vi "CollimationLightScan.vi"(6 "Backgrund":T1, 7 "Session In":T2, 10 "扫描范围":dbl) -> (2 "近场准直图像":T1(plugin-control))   [LabVIEW 2018]
uses:
  <vilib>/userdefined/High Color/IMAQdx.ctl
  <vilib>/vision/Image Controls.llb/IMAQ Image.ctl
  <vilib>/vision/NI_Vision_Development_Module.lvlib
  <vilib>/vision/driver/NI_Vision_Acquisition_Software.lvlib
  <resource>/objmgr/IMAQImage.rc
panel:
  out "offset":i32[](array[numeric])
  in  "停止":bool
  out "进度":dbl format="%05.2f%"
  out "YResolution":i32
  out "X Resolution":i32
  out "采集时间":u32
  out "运动时间":u32
  out "总时间":u32
  out "单步时间":u32
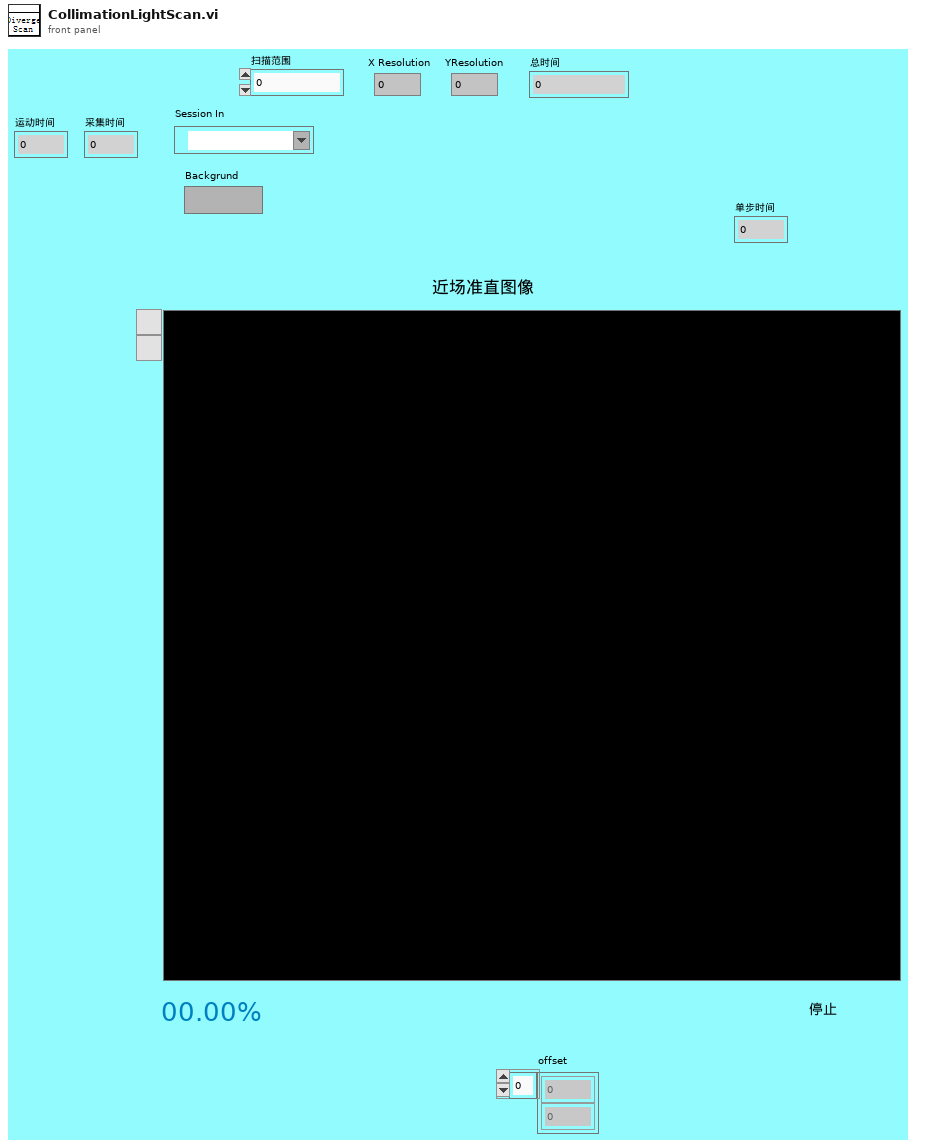
[diagram p1: front panel]
types:
  T1 = typedef "IMAQ Image.ctl" = refnum<image>
  T2 = typedef "IMAQdx.ctl" = refnum<k21>
  T3 = typedef "Image Type" = u32
  T4 = typedef "控制电机位置枚举器.ctl" = enum16{"远场扫描", "发散角扫描", "远场相机", "近场相机", "时间波形", "偏振", "能量", "功率", "光谱"}
  T5 = typedef "控制电机枚举器.ctl" = enum16{"Z", "Y", "X", "发散角", "俯仰", "旋转"}
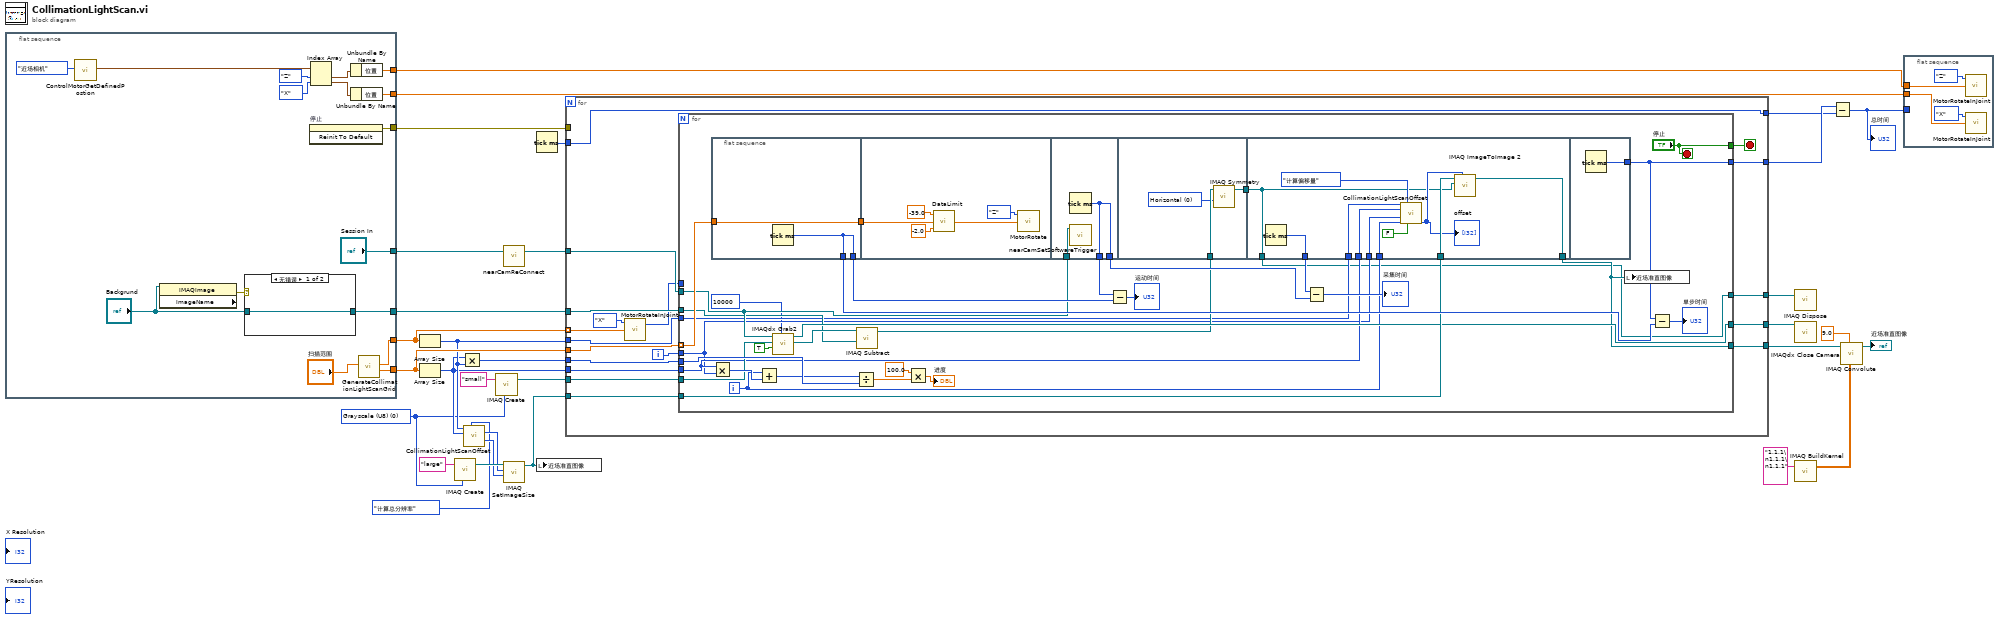
[diagram p0: block diagram]
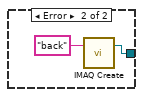
[diagram p2: hidden frame]
diagram:
  w1 = T3 0 items=["Grayscale (U8)", "Grayscale (I16)", "Grayscale (SGL)", "Complex (CSG)", "RGB (U32)", "HSL (U32)", "RGB (U64)", "Grayscale (U16)"] ("Image Type")
  n1 = flat-sequence {
    tunnel: [w35] -> w10
    tunnel: [w44] -> w31
    tunnel: [w37] -> w16
    tunnel: [w38] -> w15
    tunnel: ["Session In"] -> w13
    tunnel: [w46] -> w11
    tunnel: [w43] -> w30
    frame #0 {
      n2 = call "ControlMotorGetDefinedPostion.vi"("位置"=控制电机位置枚举器."近场相机") -> ("PosOut"=w33:cluster{"控制电机":T5, "位置":dbl}[])  [unwired: 10 in]
      n3 = property class="IMAQImage" props=["ImageName"](reference="Backgrund") -> (error out=w34:errorcluster)  [unwired: 1 in, 2 out]
      n4 = case shown="无错误" w34 {
        tunnel: "Backgrund" -> [w48 _]
        tunnel: [w48 w49] -> w35
        frame No Error {
        }
        frame Error {
          n5 = call "IMAQ Create"("Image Name"="back") -> ("New Image"=w49:T1)  [unwired: 4 in, 1 out]
        }
      }
      n6 = invoke on="停止" class="Bool" method="Reinit To Default"() -> (error out=w46:errorcluster)  [unwired: 3 in, 2 out]
      n7 = Index Array(array=w33, index #1=控制电机枚举器."Z" ("控制电机"), index #2=控制电机枚举器."X" ("控制电机")) -> (element #1=w40:cluster{"控制电机":T5, "位置":dbl}, element #2=w39:cluster{"控制电机":T5, "位置":dbl})
      n8 = Unbundle By Name(w40) -> ("位置"=w38:dbl)
      n9 = Unbundle By Name(w39) -> ("位置"=w37:dbl)
      n10 = call "GenerateCollimationLightScanGrid.vi"("扫描范围"="扫描范围") -> ("纵向扫描位置"=w43:dbl[], "横向扫描位置"=w44:dbl[])  [unwired: 9 in]
    }
  }
  n11 = Array Size(array=w31) -> (size(s)=w9:i32)
  n12 = Array Size(array=w30) -> (size(s)=w8:i32)
  n13 = call "IMAQ Create"("Image Name"="large", "Image Type"=w1) -> ("New Image"=w29:T1)  [unwired: 3 in, 1 out]
  n14 = Multiply(x=w8, y=w9) -> (x*y=w14:i32)
  n15 = call "CollimationLightScanOffset.vi"("X Pos Num"=w9, "状态"=enum16{"计算总分辨率", "计算偏移量"}."计算总分辨率", "Y Pos Num"=w8) -> ("X Resolution"=w7:i32, "Y Resolution"=w6:i32)  [unwired: 10 in, 1 out]
  n16 = call "IMAQ Create"("Image Name"="small", "Image Type"=w1) -> ("New Image"=w3:T1)  [unwired: 3 in, 1 out]
  n17 = call "nearCamReConnect.vi"("Session In"=w13) -> ("IMAQdx Session Out"=w12:T2)  [unwired: 1 in, 1 out]
  n18 = call "IMAQ SetImageSize"("Y Resolution"=w6, "X Resolution"=w7, "Image"=w29) -> ("Image Out"=w19:T1)  [unwired: 2 in, 1 out]
  n19 = Tick Count (ms)() -> (millisecond timer value=w27:u32)
  n20 = local write "近场准直图像"(w19) -> ()
  n21 = for {
    tunnel: w31 -> [w53] mode=indexing
    tunnel: w30 -> [w61]
    tunnel: w19 -> [w56]
    tunnel: w9 -> [w68]
    tunnel: w27 -> [w66]
    tunnel: [w67] -> w26
    tunnel: [w66] -> w25
    tunnel: [w65] -> w21
    tunnel: w3 -> [w64]
    tunnel: [w63] -> w18
    tunnel: w12 -> [w62]
    tunnel: w14 -> [w59]
    tunnel: w8 -> [w57]
    tunnel: w11 -> [_]
    tunnel: w10 -> [w55]
    tunnel: [w51] -> w2
    i -> [w58]
    stop <- w60 stop-if-true
    n22 = call "MotorRotateInJoint.vi"("位置"=w53, "axis"=控制电机枚举器."X" ("控制电机")) -> ("返回"=w52:i32)  [unwired: 2 in]
    n23 = for {
      tunnel: w68 -> [w75]
      tunnel: [w70] -> w65
      tunnel: [w100] -> w67
      tunnel: w64 -> [w80]
      tunnel: [w81] -> w63
      tunnel: w61 -> [w92] mode=indexing
      tunnel: ["停止"] -> w60
      tunnel: w59 -> [w90]
      tunnel: w58 -> [w73]
      tunnel: w57 -> [w74]
      tunnel: w62 -> [w82]
      tunnel: w56 -> [w84]
      tunnel: w55 -> [w77]
      tunnel: w52 -> [_]
      tunnel: [w69] -> w51
      i -> [w72]
      stop <- "停止" stop-if-true
      n24 = flat-sequence {
        tunnel: w92 -> [w104]
        tunnel: [w104] -> w102
        tunnel: [w103] -> w101
        tunnel: [w103] -> w97
        tunnel: w102 -> [w108]
        tunnel: [w111] -> w98
        tunnel: [w111] -> w94
        tunnel: w82 -> [w110]
        tunnel: w78 -> [w114]
        tunnel: [w113] -> w76
        tunnel: [w125] -> w95
        tunnel: w84 -> [w124]
        tunnel: [w123] -> w70
        tunnel: w76 -> [w115]
        tunnel: w75 -> [w121]
        tunnel: w74 -> [w120]
        tunnel: w73 -> [w119]
        tunnel: w72 -> [w118]
        tunnel: [w115] -> w69
        tunnel: [w126] -> w100
        frame #0 {
          n25 = Tick Count (ms)() -> (millisecond timer value=w103:u32)
        }
        frame #1 {
          n26 = call "DataLimit.vi"("Max"=-2.0 ("Min"), "Data"=w108, "Min"=-39.0 ("Max")) -> ("Data Out"=w107:dbl)  [unwired: 2 in]
          n27 = call "MotorRotate.vi"("位置"=w107, "控制电机"=控制电机枚举器."Z") -> ()  [unwired: 2 in, 1 out]
        }
        frame #2 {
          n28 = Tick Count (ms)() -> (millisecond timer value=w111:u32)
          n29 = call "nearCamSetSoftwareTrigger.vi"("IMAQdx Session"=w110) -> ()  [unwired: 3 in, 2 out]
        }
        frame #3 {
          w112 = u32 0 items=["Horizontal", "Vertical", "Central", "1st Diagonal", "2nd Diagonal"] ("Type of Symmetry")
          n30 = call "IMAQ Symmetry"("Type of Symmetry"=w112, "Image Src"=w114) -> ("Image Dst Out"=w113:T1)  [unwired: 3 in, 1 out]
        }
        frame #4 {
          n31 = Tick Count (ms)() -> (millisecond timer value=w125:u32)
          n32 = call "CollimationLightScanOffset.vi"("X Pos Num"=w121, "状态"=enum16{"计算总分辨率", "计算偏移量"}."计算偏移量", "Y Pos Num"=w120, "当前X位置"=w119, "当前Y位置"=w118, "正序？"=FALSE) -> ("offset"=w117:i32[])  [unwired: 7 in, 2 out]
          "offset" <- w117
          n33 = call "IMAQ ImageToImage 2"("Offset Left/Top"=w117, "Image Src (Small)"=w115, "Image Src (Large)"=w124) -> ("Image Dst Out"=w123:T1)  [unwired: 7 in, 1 out]
        }
        frame #5 {
          n34 = Tick Count (ms)() -> (millisecond timer value=w126:u32)
        }
      }
      n35 = Multiply(x=w74, y=w73) -> (x*y=w89:i32)
      n36 = Add(x=w72, y=w89) -> (x+y=w88:i32)
      n37 = call <vilib>:"IMAQdx Grab2.vi"("Timeout (ms)"=10000, "Wait for Next Buffer? (Yes)"=TRUE, "Image In"=w80, "Session In"=w82) -> ("Image Out"=w79:T1, "Session Out"=w81:T2)  [unwired: 4 in, 2 out]
      n38 = Divide(x=w88, y=w90) -> (x/y=w87:dbl)
      n39 = call "IMAQ Subtract"("Image Src A"=w79, "Image Src B"=w77) -> ("Image Dst Out"=w78:T1)  [unwired: 5 in, 1 out]
      n40 = Multiply(x=100.0, y=w87) -> (x*y=→"进度":dbl)
      n41 = Subtract(x=w98, y=w97) -> (x-y=→"运动时间":u32)
      n42 = Subtract(x=w95, y=w94) -> (x-y=→"采集时间":u32)
      n43 = local write "近场准直图像"(w70) -> ()
      n44 = Subtract(x=w100, y=w101) -> (x-y=→"单步时间":u32)
    }
  }
  n45 = call "IMAQ Dispose"("Image"=w2) -> ()  [unwired: 5 in, 1 out]
  n46 = call <vilib>:"IMAQdx Close Camera.vi"("Session In"=w18) -> ()  [unwired: 10 in, 1 out]
  n47 = call "IMAQ BuildKernel"("Kernel String"="1,1,1\n1,1,1\n1,1,1") -> ("Kernel"=w22:sgl[][])  [unwired: 4 in, 1 out]
  n48 = Subtract(x=w26, y=w25) -> (x-y=w17:u32)
  "总时间" <- w17
  n49 = call "IMAQ Convolute"("Kernel"=w22, "Divider (kernel sum)"=sgl 9.0, "Image Src"=w21) -> ("Image Dst Out"=→"近场准直图像":T1)  [unwired: 7 in, 1 out]
  n50 = flat-sequence {
    tunnel: w17 -> [_]
    tunnel: w16 -> [w128]
    tunnel: w15 -> [w127]
    frame #0 {
      n51 = call "MotorRotateInJoint.vi"("位置"=w127, "axis"=控制电机枚举器."Z" ("控制电机")) -> ()  [unwired: 2 in, 1 out]
      n52 = call "MotorRotateInJoint.vi"("位置"=w128, "axis"=控制电机枚举器."X" ("控制电机")) -> ()  [unwired: 2 in, 1 out]
    }
  }
